vi "NetComm_UnloadCPPStartupProgram.vi"(8 "error in (no error)":errorcluster) -> (0 "error out":errorcluster, 2 "return code":i32)   [LabVIEW 2017]
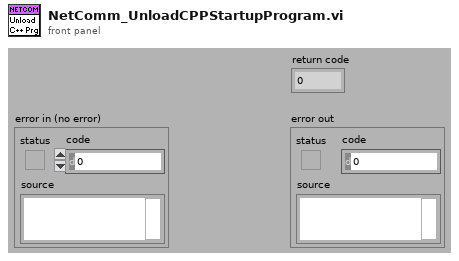
[diagram p1: front panel]
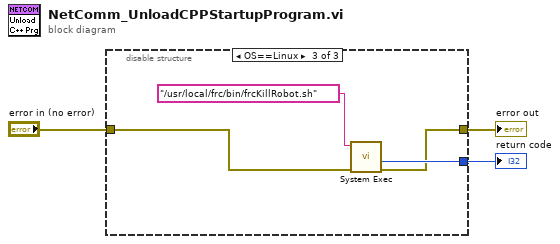
[diagram p0: block diagram]
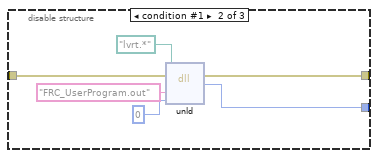
[diagram p3: hidden frame]
diagram:
  n1 = disable-structure shown="OS==Linux" {
    disable-tunnel: "error in (no error)" -> [w4 w8 w11]
    disable-tunnel: [w4 w7 w12] -> w2
    disable-tunnel: [_ w6 w13] -> w1
    frame condition #0 {
    }
    frame condition #1 {
      n2 = dll-call lib="?" fn="unld" ("LabVIEW.dll:printf")(path in=path "lvrt.*", error in=w8, "module"="FRC_UserProgram.out" ("format"), "options"=0) -> (error out=w7:errorcluster, "return type"=w6:i32)  [unwired: 2 in, 2 out]
    }
    frame condition #2 (active) {
      n3 = call <vilib>:"System Exec.vi"("error in (no error)"=w11, "command line"="/usr/local/frc/bin/frcKillRobot.sh") -> ("error out"=w12:errorcluster, "return code"=w13:i32)  [unwired: 6 in, 2 out]
    }
  }
  "error out" <- w2
  "return code" <- w1
